vi "Interrogate Target.vi"(8 "Error In":errorcluster, 11 "Install LV Data":T1={"SSH Session"=refnum, "Status Log"="", "Detailed Log"="", "Credentials"={"Hostname or IP"="192.168.7.2", "Username"="root", "Password"=""}, "Target Info"={"OS Version"="", "CPU"="", "Systemd Version"="", "Internet Access"=FALSE, "Device Type"=""}, "Reboot Required?"=FALSE}) -> (0 "Error Out":errorcluster, 1 "Status":string="Unable To Interrogate The Device", 2 "Target Info":T2, 3 "Install LV Data":T1={"SSH Session"=refnum, "Status Log"="", "Detailed Log"="", "Credentials"={"Hostname or IP"="192.168.7.2", "Username"="root", "Password"=""}, "Target Info"={"OS Version"="", "CPU"="", "Systemd Version"="", "Internet Access"=FALSE, "Device Type"=""}, "Reboot Required?"=FALSE})   [LabVIEW 2014, in "LMH-LINX.lvlib"]
uses:
  LMH-LINX.lvlib
  Target Info.ctl
  Install LV Data.ctl
  C:/github/makerhub/LINX/LabVIEW/vi.lib/MakerHub/LINX/Resources/Renci.SshNet.dll
  Resources/Renci.SshNet.dll
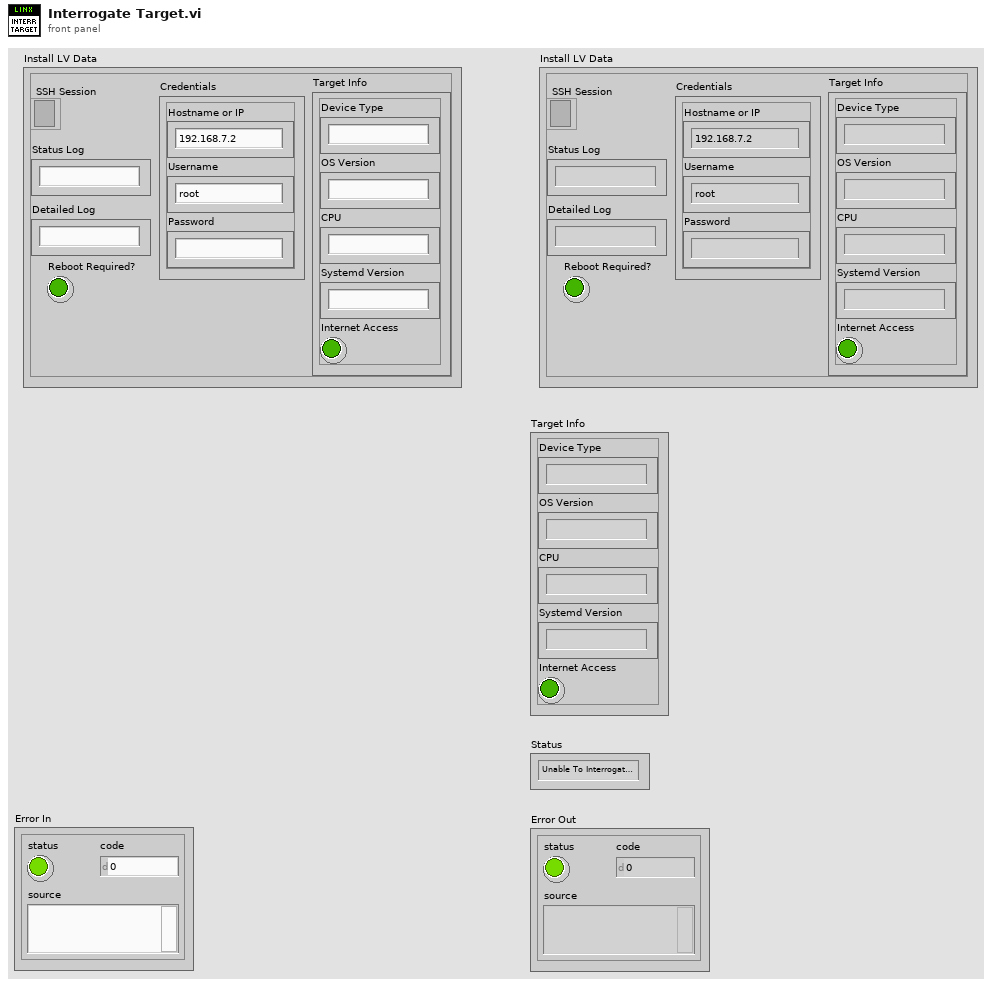
[diagram p1: front panel]
types:
  T1 = typedef "LMH-LINX.lvlib/Install LV Data.ctl" = cluster{"SSH Session":refnum<k24>, "Status Log":string, "Detailed Log":string, "Credentials":cluster{"Hostname or IP":string, "Username":string, "Password":string}, "Target Info":T2, "Reboot Required?":bool}
  T2 = typedef "LMH-LINX.lvlib/Target Info.ctl" = cluster{"OS Version":string, "CPU":string, "Systemd Version":string, "Internet Access":bool, "Device Type":string}
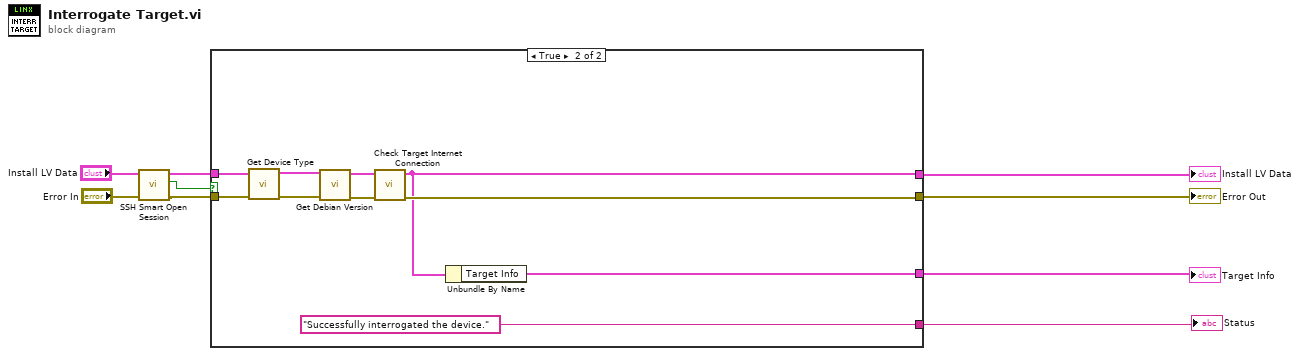
[diagram p0: block diagram]
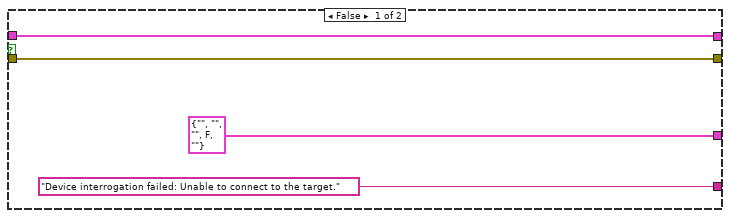
[diagram p2: hidden frame]
diagram:
  n1 = call "SSH Smart Open Session.vi"("Error In"="Error In", "Install LV Data in"="Install LV Data") -> ("Error Out"=w4:errorcluster, "Connected?"=w2:bool, "Install LV Data out"=w5:T1)  [unwired: 6 in, 1 out]
  n2 = case shown="True" w2 {
    tunnel: [T2 {"OS Version"="", "CPU"="", "Systemd Version"="", "Internet Access"=FALSE, "Device Type"=""} ("Target Info") w16] -> w9
    tunnel: [w11 w15] -> w1
    tunnel: w4 -> [w11 w22]
    tunnel: ["Device interrogation failed: Unable to connect to the target." "Successfully interrogated the device."] -> w8
    tunnel: w5 -> [w10 w20]
    tunnel: [w10 w14] -> w7
    frame False {
    }
    frame True {
      n3 = call "Get Device Type.vi"("Error In"=w22, "Install LV Data"=w20) -> ("Error Out"=w23:errorcluster, "Install LV Data"=w19:T1)  [unwired: 7 in, 1 out]
      n4 = call "Get Debian Version.vi"("Error In"=w23, "Install LV Data"=w19) -> ("Error Out"=w17:errorcluster, "Install LV Data"=w18:T1)  [unwired: 7 in, 1 out]
      n5 = call "Check Target Internet Connection.vi"("Error In"=w17, "Install LV Data"=w18) -> ("Error Out"=w15:errorcluster, "Install LV Data"=w14:T1)  [unwired: 8 in]
      n6 = Unbundle By Name(w14) -> ("Target Info"=w16:T2)
    }
  }
  "Error Out" <- w1
  "Target Info" <- w9
  "Install LV Data" <- w7
  "Status" <- w8
